vi "al_dmm_range.vi"(0 "DMM TSM In":T3, 1 "DC Voltage Range":T4(ring), 5 "Function":T2, 7 "Resolution in Digits":T1=7.5 items=["3 1/2"=3.5, "4 1/2"=4.5, "5 1/2"=5.5, "6 1/2"=6.5, "7 1/2"=7.5], 11 "error in":errorcluster, 12 "Aperture Time (s)":dbl=0.01666 format="%#_13p") -> (15 "error out":errorcluster)   [LabVIEW 2019]
doc: "This SubVI configure the settings of DMM"
uses:
  Instrument Control/DMM/Pin Map/TSM DMM.ctl
  <vilib>/NI_TestStand_SemiconductorModule/NI_TestStand_Semiconductor_Module.lvlibp/PinMap/PinQueryContext/MultiplePinMultipleSessionQueryContext/MultiplePinMultipleSessionQueryContext.lvclass
  <instrlib>/niDMM/nidmm.llb/niDMM Function.ctl
  <instrlib>/niDMM/nidmm.llb/niDMM Resolution in Digits.ctl
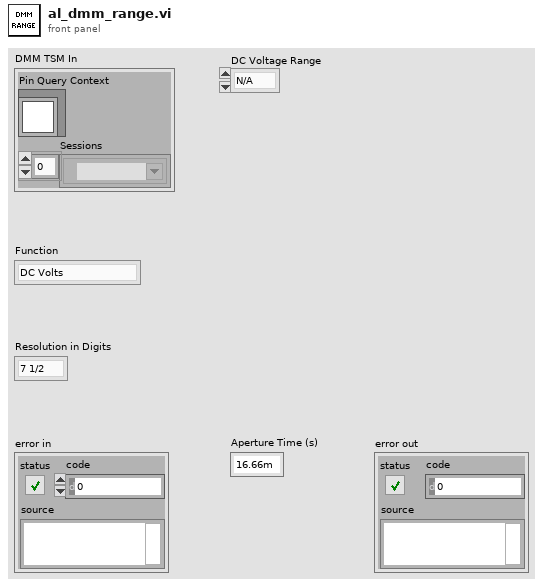
[diagram p1: front panel]
types:
  T1 = typedef "niDMM Resolution in Digits.ctl" = dbl
  T2 = typedef "niDMM Function.ctl" = enum16{"DC Volts", "AC Volts", "DC Current", "AC Current", "2-wire Resistance", "4-wire Resistance", "Diode", "Frequency", "Period", "AC Volts DC Coupled", "Capacitance", "Inductance", "Temperature"}
  T3 = typedef "TSM DMM.ctl" = cluster{"Pin Query Context":refnum<class "MultiplePinMultipleSessionQueryContext.lvclass">, "Sessions":refnum<k15>[]}
  T4 = enum16{"N/A", "100mV", "1V", "10V", "100V", "1000V"}
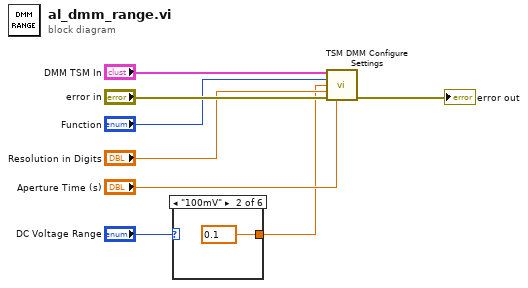
[diagram p0: block diagram]
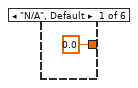
[diagram p2: hidden frame]
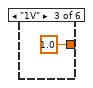
[diagram p3: hidden frame]
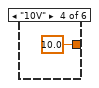
[diagram p4: hidden frame]
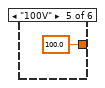
[diagram p5: hidden frame]
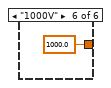
[diagram p6: hidden frame]
diagram:
  n1 = case shown="\"100mV\"" "DC Voltage Range" {
    tunnel: [0.0 ("Source:DC Current:Current Level Range") 0.1 ("Source:DC Current:Current Level Range") 1.0 ("Source:DC Current:Current Level Range") 10.0 ("Source:DC Current:Current Level Range") 100.0 ("Source:DC Current:Current Level Range") 1000.0 ("Source:DC Current:Current Level Range")] -> w1
    frame "N/A", Default {
    }
    frame "100mV" {
    }
    frame "1V" {
    }
    frame "10V" {
    }
    frame "100V" {
    }
    frame "1000V" {
    }
  }
  n2 = call "TSM DMM Configure Settings.vi"("DMM TSM In"="DMM TSM In", "Function"="Function", "Range"=w1, "Resolution in Digits"="Resolution in Digits", "error in"="error in", "Aperture Time (s)"="Aperture Time (s)") -> ("error out"=→"error out":errorcluster)  [unwired: 8 in, 1 out]
